vi "TempToAtmel.vi"(11 "TempSP":dbl) -> (3 "ToAtmel":dbl)   [LabVIEW 2020]
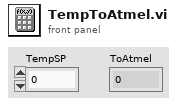
[diagram p1: front panel]
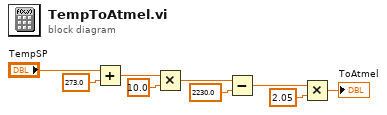
[diagram p0: block diagram]
diagram:
  n1 = Add(x="TempSP", y=273.0) -> (x+y=w6:dbl)
  n2 = Multiply(x=w6, y=10.0) -> (x*y=w8:dbl)
  n3 = Subtract(x=w8, y=2230.0 ("x")) -> (x-y=w3:dbl)
  n4 = Multiply(x=w3, y=2.05 ("x")) -> (x*y=→"ToAtmel":dbl)
